vi "Single Data.vi"   [LabVIEW 2010]
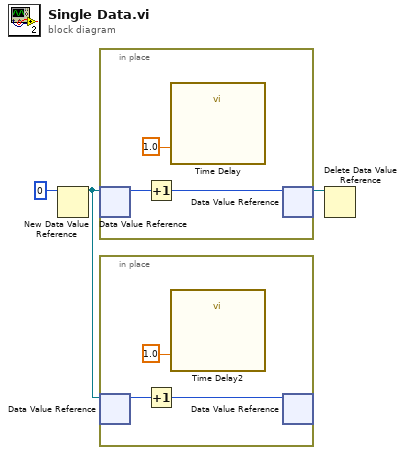
[diagram p0: block diagram]
diagram:
  n1 = New Data Value Reference(data value=0) -> (data value reference=w1:refnum<data-value>)  [unwired: 1 in, 1 out]
  n2 = in-place {
    n3 = in-place-dvr #1(w1) -> (w6:i32)  [unwired: 1 out]
    n4 = Increment(x=w6) -> (x+1=w5:i32)
    n5 = call "Time Delay"("Delay Time (s)"=1.0) -> ()  [unwired: 10 in, 1 out]
    n6 = in-place-dvr #1(w5) -> (w2:refnum<data-value>)  [unwired: 1 out]
  }
  n7 = in-place {
    n8 = in-place-dvr #2(w1) -> (w9:i32)  [unwired: 1 out]
    n9 = Increment(x=w9) -> (x+1=w8:i32)
    n10 = call "Time Delay2"("Delay Time (s)"=1.0) -> ()  [unwired: 10 in, 1 out]
    n11 = in-place-dvr #2(w8) -> ()  [unwired: 2 out]
  }
  n12 = Delete Data Value Reference(data value reference=w2) -> ()  [unwired: 1 in, 2 out]
